vi "ReadChannelList.vi"(8 "error in":errorcluster, 11 "DAQ ID #":i32) -> (0 "error out":errorcluster, 3 "Read Channels":string)   [LabVIEW 2024]
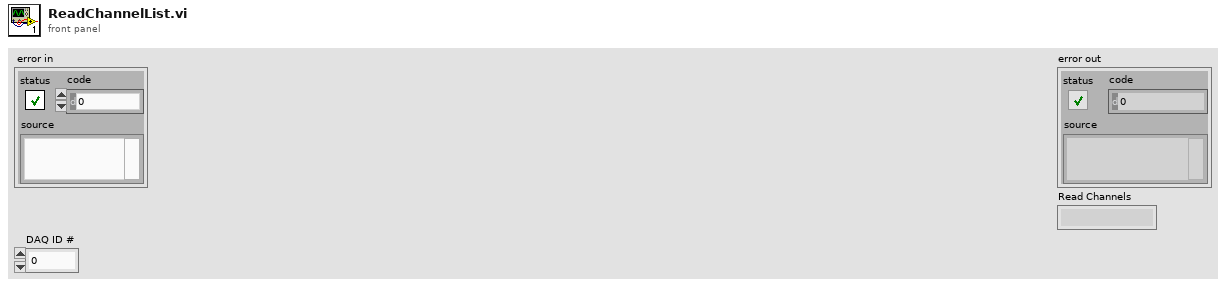
[diagram p1: front panel]
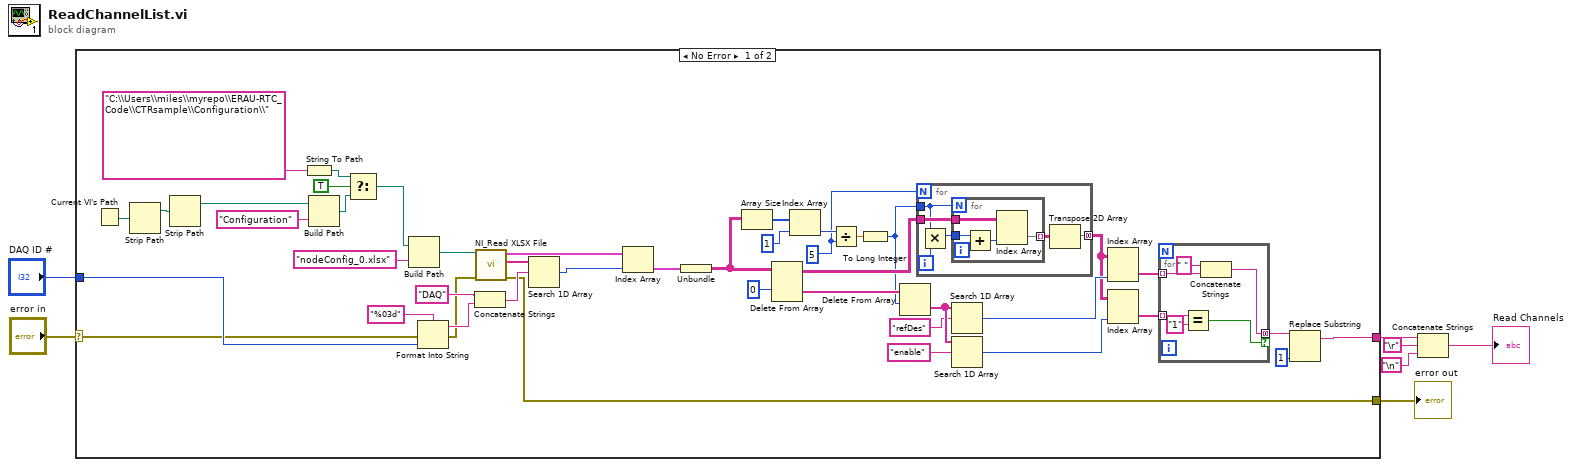
[diagram p0: block diagram]
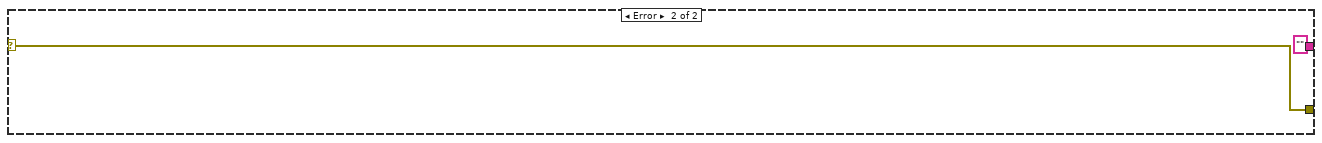
[diagram p2: hidden frame]
diagram:
  n1 = case shown="No Error" "error in" {
    selector: "error in" -> [w30 w69]
    tunnel: "DAQ ID #" -> [w36 _]
    tunnel: [w13 ""] -> w2
    tunnel: [w29 w69] -> w5
    frame No Error {
      w22 = 5 ("y")
      n2 = Current VI's Path() -> (path=w49:path)
      n3 = Strip Path(path=w49) -> (stripped path=w47:path)  [unwired: 1 out]
      n4 = Strip Path(path=w47) -> (stripped path=w46:path)  [unwired: 1 out]
      n5 = String To Path(string="C:\\Users\\miles\\myrepo\\ERAU-RTC_Code\\CTRsample\\Configuration\\") -> (path=w9:path)
      n6 = Build Path(base path=w46, name or relative path="Configuration") -> (appended path=w12:path)
      n7 = Select(t=w9, s=TRUE, f=w12) -> (s? t:f=w11:path)
      n8 = Build Path(base path=w11, name or relative path="nodeConfig_0.xlsx") -> (appended path=w50:path)
      n9 = Format Into String(format string="%03d", error in=w30, w36) -> (resulting string=w40:string, error out=w38:errorcluster)  [unwired: 1 in]
      n10 = Concatenate Strings("DAQ" ("string"), w40) -> (w42:string)
      n11 = call "NI_Read XLSX File.vi"("error in"=w38, "XLSX File"=w50) -> ("error out"=w29:errorcluster, "Sheet Names"=w43:string[], "Sheet Data"=w45:cluster{"Array":string[][]}[])  [unwired: 7 in]
      n12 = Search 1D Array(1D array=w43, element=w42) -> (index of element=w37:i32)  [unwired: 1 in]
      n13 = Index Array(array=w45, index=w37) -> (element=w44:cluster{"Array":string[][]})
      n14 = Unbundle(w44) -> ("Array"=w28:string[][])
      n15 = Array Size(array=w28) -> (size(s)=w35:i32[])
      n16 = Delete From Array(array=w28, index (row)=0) -> (deleted portion=w24:string[], array with subset deleted=w23:string[][])  [unwired: 2 in]
      n17 = Index Array(array=w35, index=1) -> (element=w33:i32)
      n18 = Divide(x=w33, y=w22) -> (x/y=w31:dbl)
      n19 = To Long Integer(number=w31) -> (32bit integer=w21:i32)
      n20 = Delete From Array(array=w24, length=w21) -> (deleted portion=w27:string[])  [unwired: 1 in, 1 out]
      n21 = for {
        N: w22 -> [_]
        tunnel: w23 -> [w63]
        tunnel: w21 -> [w61]
        tunnel: [w58] -> w19 mode=concatenating
        i -> [w62]
        n22 = Multiply(x=w61, y=w62) -> (x*y=w60:i32)
        n23 = for {
          N: w61 -> [_]
          tunnel: w63 -> [w68]
          tunnel: w60 -> [w66]
          tunnel: [w64] -> w59 mode=indexing
          i -> [w67]
          n24 = Add(x=w66, y=w67) -> (x+y=w65:i32)
          n25 = Index Array(array=w68, index (col)=w65) -> (element=w64:string[])  [unwired: 1 in]
        }
        n26 = Transpose 2D Array(2D array=w59) -> (transposed array=w58:string[][])
      }
      n27 = Search 1D Array(1D array=w27, element="refDes") -> (index of element=w20:i32)  [unwired: 1 in]
      n28 = Search 1D Array(1D array=w27, element="enable") -> (index of element=w18:i32)  [unwired: 1 in]
      n29 = Index Array(array=w19, index (col)=w20) -> (element=w17:string[])  [unwired: 1 in]
      n30 = Index Array(array=w19, index (col)=w18) -> (element=w16:string[])  [unwired: 1 in]
      n31 = for {
        tunnel: w17 -> [w57] mode=indexing
        tunnel: w16 -> [w54] mode=indexing
        tunnel: [w56] -> w15 mode=concatenating if=w52
        n32 = Equal?(x=w54, y="1") -> (x = y?=w52:bool)
        n33 = Concatenate Strings(" " ("string"), w57) -> (w56:string)
      }
      n34 = Replace Substring(2:1 ("length (len. of substring)"), 5:w15) -> (1:w13:string)  [unwired: 2 in, 1 out]
    }
    frame Error {
    }
  }
  "error out" <- w5
  n35 = Concatenate Strings(w2, "\r", "\n") -> (→"Read Channels":string)
